vi "载荷控制(3).vi"() -> ()   [LabVIEW 2020]
doc: "The Basic Serial Read and Write example performs a Serial Port Read, a Serial Port Write, or a combination of these actions. The user selects the actions (read or write) on the front panel. If both are selected, the VI will write the data first, read data, and then close the VISA session that is opened to the port. This VI will wait until the specified number of bytes is received at the port. Only the number of bytes specified will be read.\n\nINSTRUCTIONS:\n1) Select the serial resource and configuration parameters (baud rate, data bits, parity, stop bits, flow control).\n2) Select the operations to be performed. \n3) Connect the serial port to your device. If no device is available, perform a loopback test by doing one of the following. Short pins 2 and 3 on a RS-232 cable or short pin 4 to pin 8 and pin 5 to pin 9 on a RS-485/422 cable. \n4) Run the VI to see the data read. (The \"read string\" will match the \"string to write\" if a loopback test was performed.)\n\nNote: The parameters set for the serial port must match the parameters of the connected instrument or device. In this example, the bytes to read parameter specifies the number of bytes that the serial port reads. If there were more bytes at the port than the number specified in bytes to read, those bytes would not be read. Also, if you specify to read more bytes than the number of bytes actually read, you might receive a timeout error message.\n\nOn the block diagram, the Configure Serial Port VI sets the configuration parameters. The front panel displays the controls used to configure the basic parameters, such as baud rate, data bits, and parity. Constants configure the other parameters the user probably does not need set. After the VISA Configure Serial Port VI opens the VISA session and configures the port, the VI passes the VISA resource name to other VIs that perform operations on that VISA resource. The VISA Write function sends a command to the serial device and the VISA Read function returns data based on the command. The VISA Close function then closes the reference to the serial device. It is important to close the reference; otherwise communication through with that port through protocols other than VISA might not be possible."
uses:
  <vilib>/Analysis/baseanly.llb/Mean (DBL).vi
  <vilib>/Instr/_visa.llb/VISA Configure Serial Port (Instr).vi
  <vilib>/Analysis/NI_AALBase.lvlib
panel:
  in  "停止 3":bool
  out "位移(微米）":dbl format="%#.2f"
  out "数据":dbl
  out "原始载荷":dbl format="%#.2f"
  out "当前次数":i32
  in  "选项卡控件":enum32{"设置", "手动", "自动", "循环加载"}(tab)
  in  "设置串口":refnum<visa-resource-name>="COM1"
  in  "载荷测量":tag="cDAQ9184-1ADFF13Mod3"
  in  "气流控制":tag="Dev2"
  in  "?":bool
  in  "?":bool
  in  "?":bool
  in  "?":bool
  in  "位置清零":bool
  in  "载荷清零":bool
  in  "加载":bool
  in  "比例系数":i32 min=0 max=1000
  in  "设定载荷":i32 min=0 max=1000
  in  "形变速率（微米/秒）":i32 min=0
  in  "火焰控制":dbl format="%#_6f"
  in  "冷却控制":dbl
  in  "开":bool
  in  "低载时间":dbl
  in  "高载时间":dbl
  in  "低载荷":dbl
  in  "高载荷":dbl
  in  "循环次数":i32
  out "载荷（牛）":dbl format="%.2f"
  out "载荷零点\n（牛）":dbl
  in  "停止":bool
  out "拉压":dbl
  in  "触发":u8
  out "结果":i16
  in  "实际位置":i32
  out "位移(微米）":dbl
  in  "停止 2":bool
  in  "自动\n\n手动":bool
  # "微调"
  # "粗调"
  # "关"
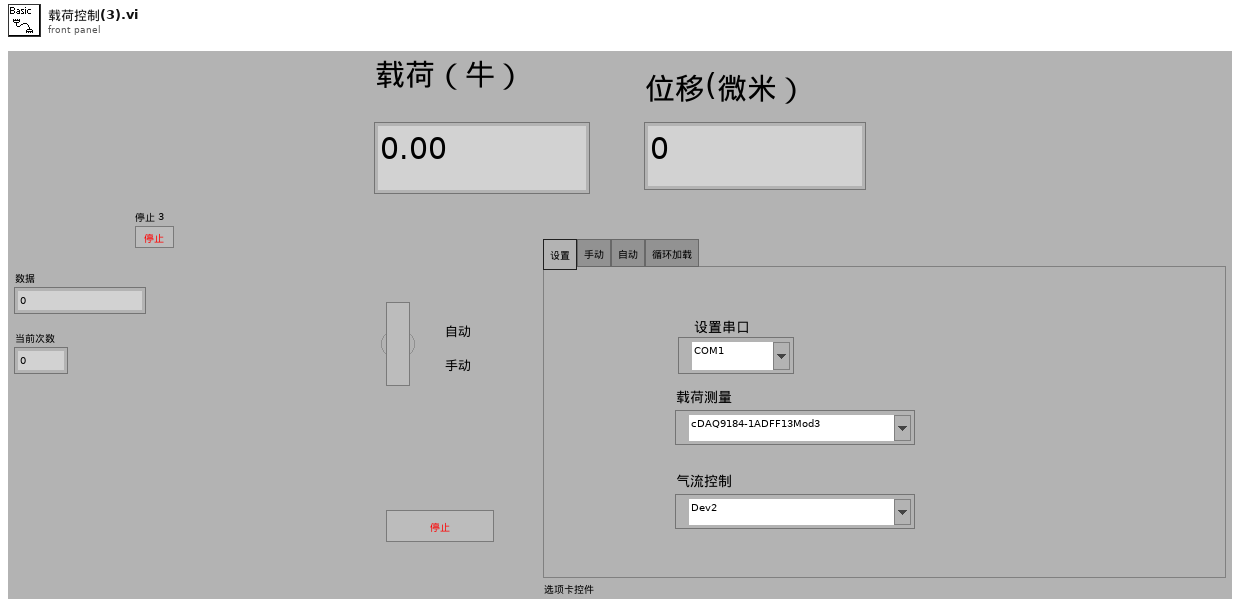
[diagram p1: front panel]
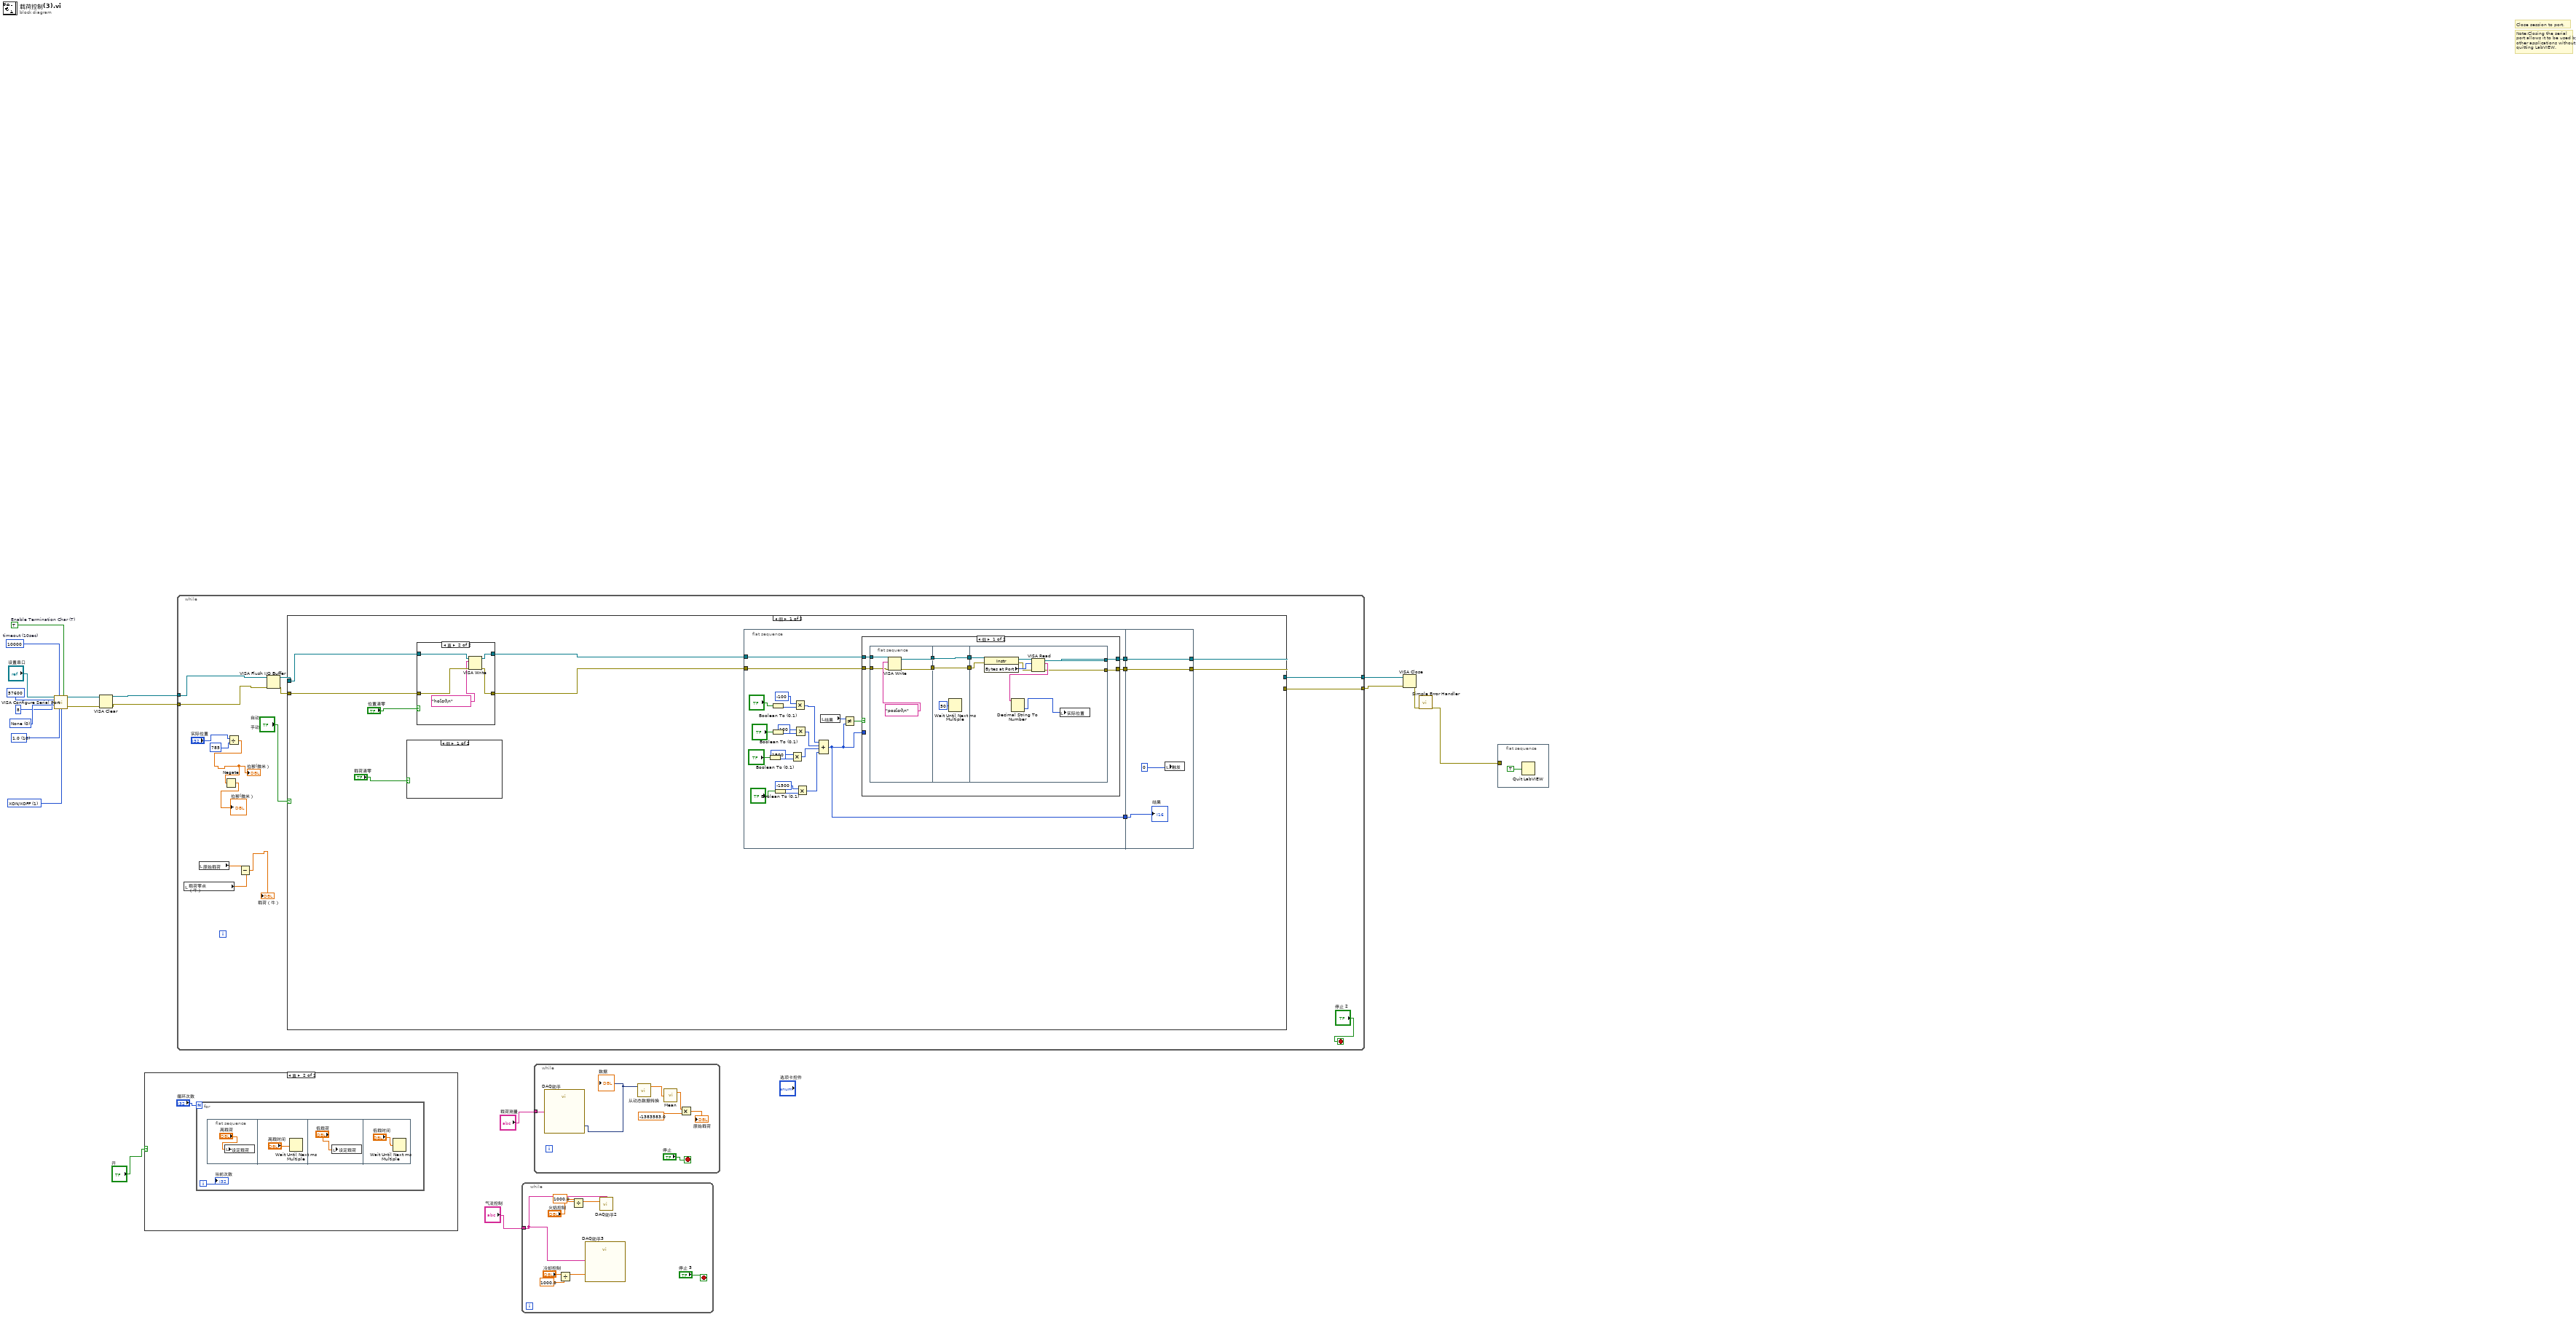
[diagram p0: block diagram]
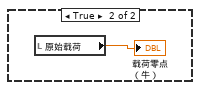
[diagram p3: hidden frame]
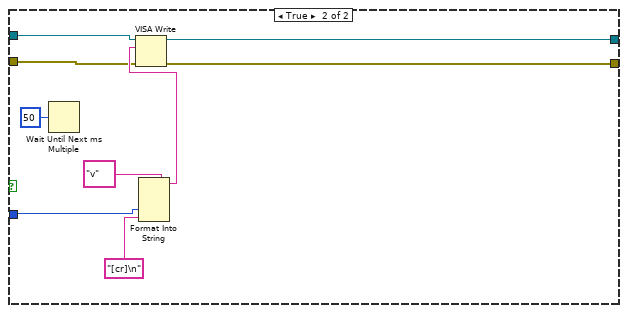
[diagram p5: hidden frame]
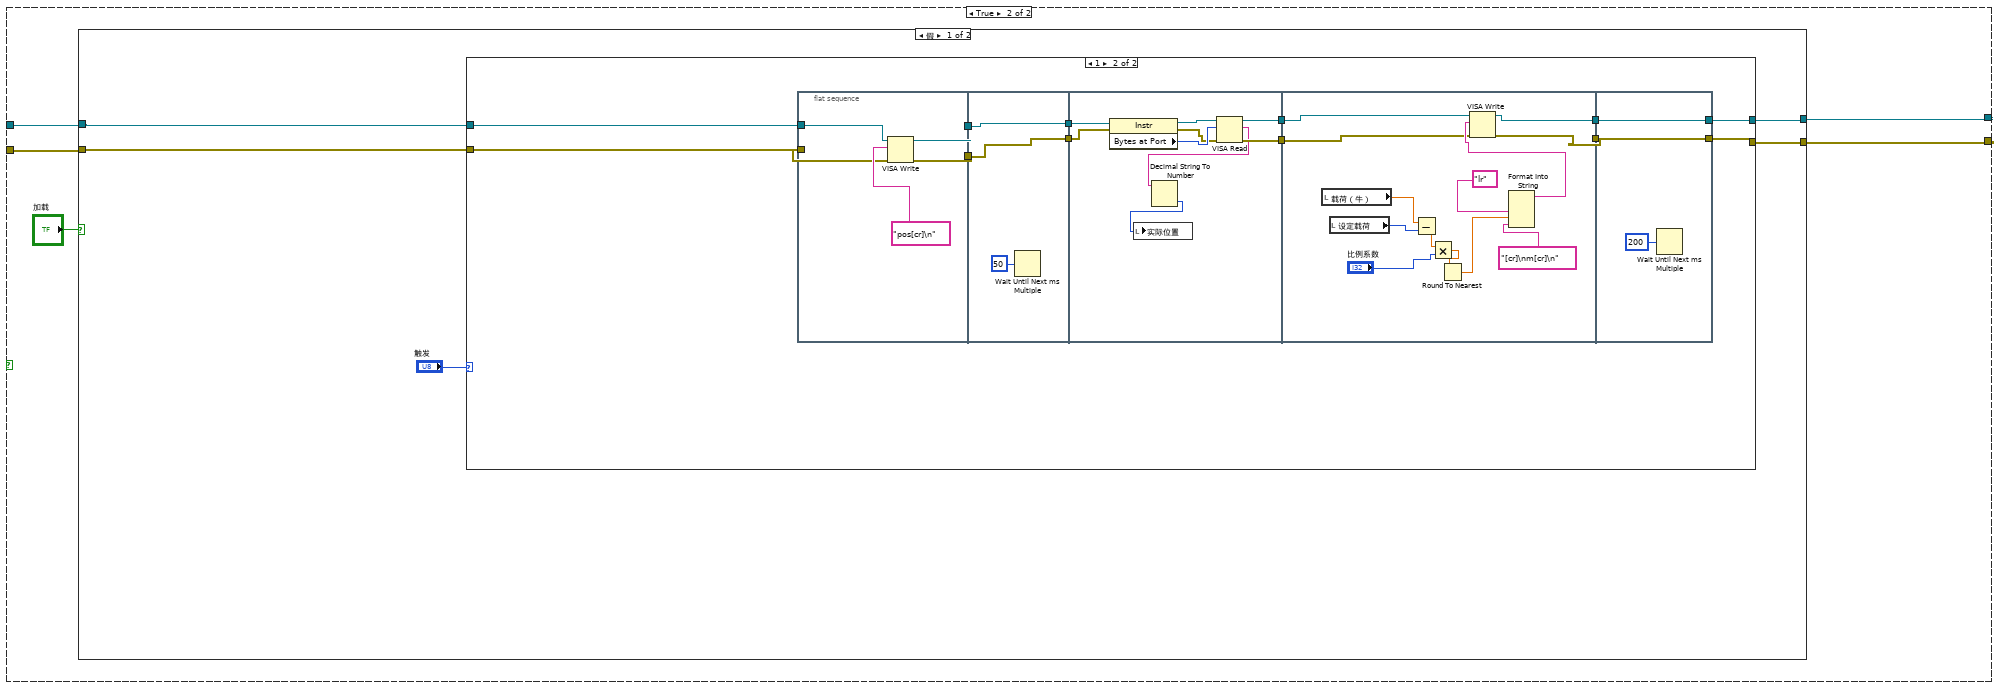
[diagram p6: hidden frame]
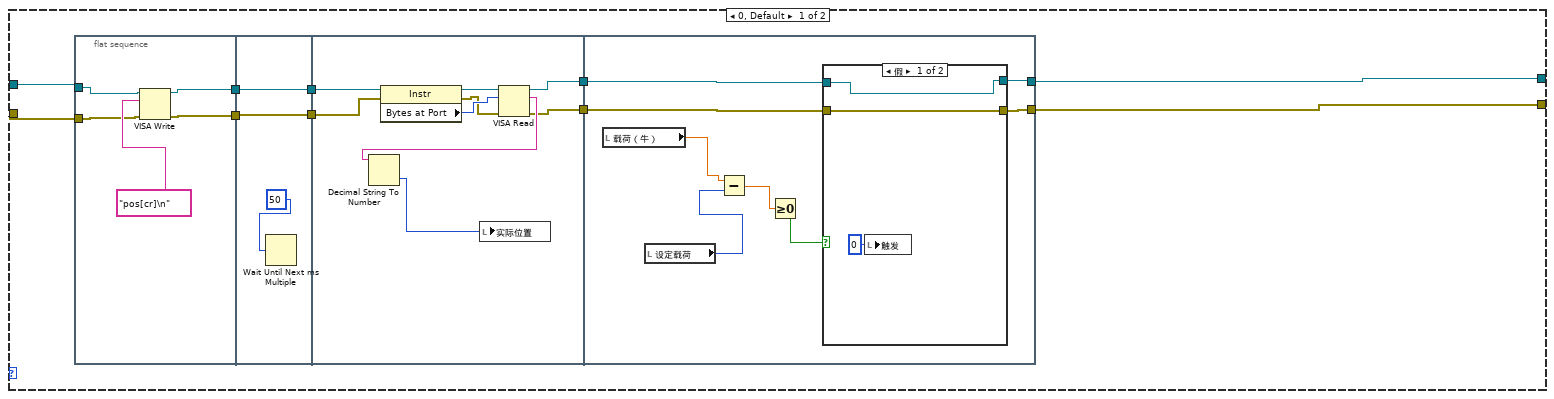
[diagram p7: hidden frame]
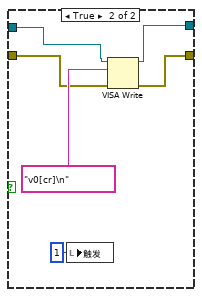
[diagram p8: hidden frame]
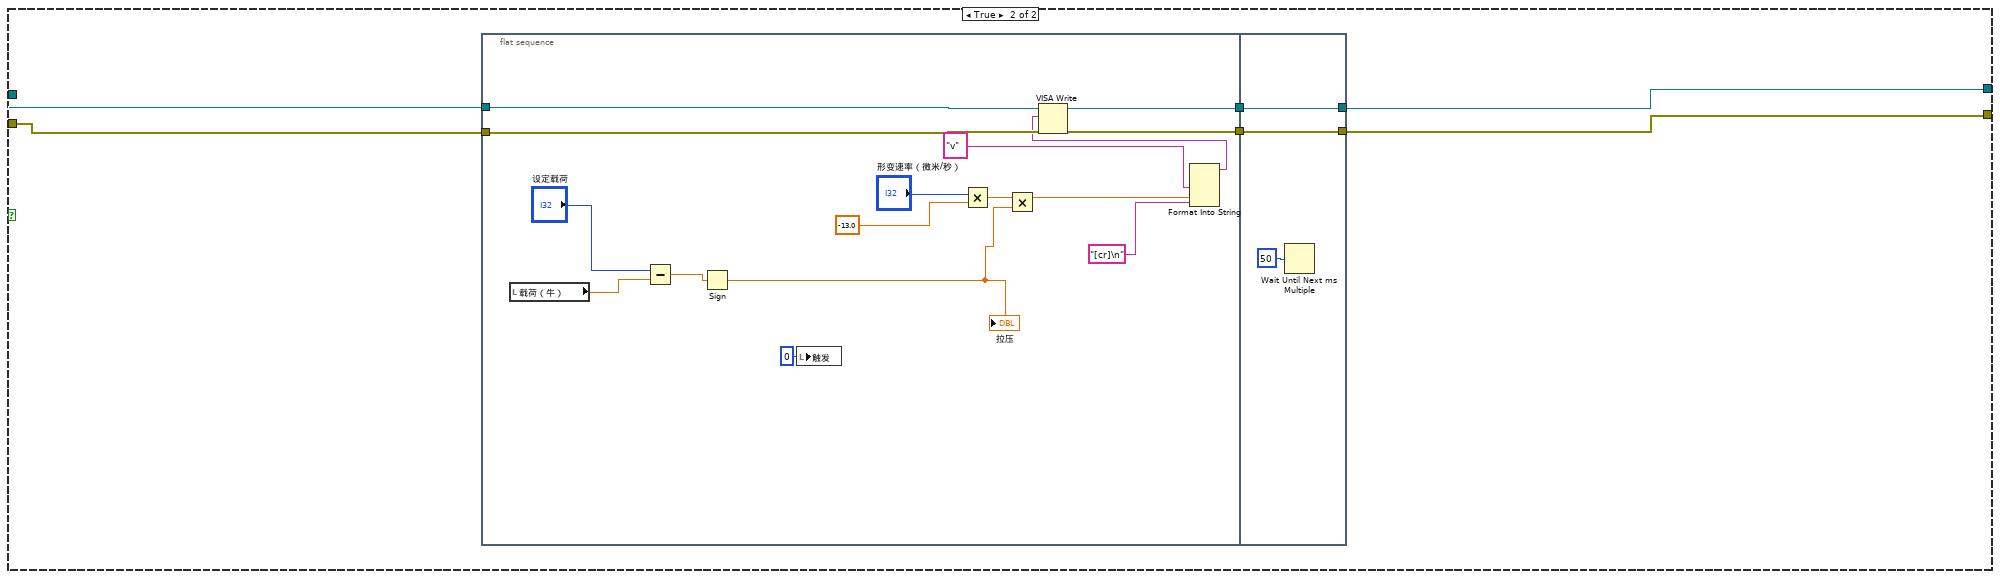
[diagram p9: hidden frame]
diagram:
  w13 = u16 1 items=["None"=0, "XON/XOFF"=1, "RTS/CTS"=2, "DTR/DSR"=4] ("flow control")
  w14 = u16 10 items=["1.0"=10, "1.5"=15, "2.0"=20] ("stop bits")
  w17 = u16 0 items=["None", "Odd", "Even", "Mark", "Space"] ("parity")
  w15 = TRUE  # Enable Termination Char (T)
  w16 = u32 10000  # timeout (10sec)
  # "Note:Closing the serial port allows it to be used by other applications without\nquitting LabVIEW."
  # "Close session to port."
  n1 = call-poly "VISA Configure Serial Port"("VISA resource name"="设置串口", "timeout (10sec)"=w16, "Enable Termination\nChar (T)"=w15, "baud rate (9600)"=u32 57600 ("baud rate"), "data bits (8)"=u16 8 ("data bits"), "parity (0:none)"=w17, "stop bits (10: 1 bit)"=w14, "flow control (0:none)"=w13) -> ("VISA resource name out"=w5:refnum<visa-resource-name>, "error out"=w7:errorcluster)  [unwired: 6 in]
  n2 = VISA Clear(VISA resource name=w5, error in (no error)=w7) -> (VISA resource name out=w6:refnum<visa-resource-name>, error out=w8:errorcluster)
  n3 = case shown="真" "开" {
    frame False {
    }
    frame True {
      n4 = for {
        N: "循环次数" -> [_]
        i -> [w21]
        n5 = flat-sequence {
          frame #0 {
            n6 = local write "设定载荷"("高载荷") -> ()
          }
          frame #1 {
            n7 = Wait Until Next ms Multiple(millisecond multiple="高载时间") -> ()  [unwired: 1 out]
          }
          frame #2 {
            n8 = local write "设定载荷"("低载荷") -> ()
          }
          frame #3 {
            n9 = Wait Until Next ms Multiple(millisecond multiple="低载时间") -> ()  [unwired: 1 out]
          }
        }
        "当前次数" <- w21
      }
    }
  }
  n10 = while {
    tunnel: w6 -> [w31]
    tunnel: w8 -> [w32]
    tunnel: [w38] -> w10
    tunnel: [w37] -> w9
    stop <- "停止 2" stop-if-true
    n11 = local read "载荷零点\n（牛）"() -> (w29:dbl)
    n12 = local read "原始载荷"() -> (w30:dbl)
    n13 = Divide(x="实际位置", y=785) -> (x/y=w26:dbl)
    "位移(微米）" <- w26
    n14 = Negate(x=w26) -> (-x=→"位移(微米）":dbl)
    n15 = Subtract(x=w30, y=w29) -> (x-y=→"载荷（牛）":dbl)
    n16 = VISA Flush I/O Buffer(VISA resource name=w31, error in (no error)=w32) -> (VISA resource name out=w34:refnum<visa-resource-name>, error out=w33:errorcluster)  [unwired: 1 in]
    n17 = case shown="假" "自动\n\n手动" {
      tunnel: w34 -> [w46 w125]
      tunnel: w33 -> [w44 w121]
      tunnel: [w48 w123] -> w38
      tunnel: [w47 w122] -> w37
      frame False {
        n18 = case shown="假" "载荷清零" {
          frame False {
          }
          frame True {
            n19 = local read "原始载荷"() -> (→"载荷零点\n（牛）":dbl)
          }
        }
        n20 = case shown="真" "位置清零" {
          tunnel: w46 -> [w54 w59]
          tunnel: [w54 w58] -> w45
          tunnel: w44 -> [w53 w57]
          tunnel: [w53 w56] -> w43
          frame False {
          }
          frame True {
            n21 = VISA Write(VISA resource name=w59, write buffer="ho[cr]\n" ("输入 1"), error in (no error)=w57) -> (VISA resource name out=w58:refnum<visa-resource-name>, error out=w56:errorcluster)  [unwired: 1 out]
          }
        }
        n22 = flat-sequence {
          tunnel: [w82] -> w51
          tunnel: [w69] -> w49
          tunnel: [w68] -> w50
          tunnel: w45 -> [w65]
          tunnel: w43 -> [w66]
          tunnel: w51 -> [w119]
          tunnel: w50 -> [w120]
          tunnel: w49 -> [w118]
          tunnel: [w119] -> w48
          tunnel: [w118] -> w47
          frame #0 {
            n23 = Boolean To (0,1)(Boolean="?") -> (0, 1=w62:i16)
            n24 = Boolean To (0,1)(Boolean="?") -> (0, 1=w80:i16)
            n25 = Boolean To (0,1)(Boolean="?") -> (0, 1=w78:i16)
            n26 = Boolean To (0,1)(Boolean="?") -> (0, 1=w76:i16)
            n27 = Multiply(x=i16 1500, y=w62) -> (x*y=w60:i16)
            n28 = Multiply(x=i16 -100, y=w80) -> (x*y=w73:i16)
            n29 = Multiply(x=i16 100, y=w78) -> (x*y=w72:i16)
            n30 = Multiply(x=i16 -1500, y=w76) -> (x*y=w71:i16)
            n31 = Compound Arithmetic op=ADD(w73, w72, w60, w71) -> (w68:i16)
            n32 = local read "结果"() -> (w67:i16)
            n33 = Not Equal?(x=w67, y=w68) -> (x != y?=w70:bool)
            n34 = case shown="假" w70 {
              tunnel: w65 -> [w86 w110]
              tunnel: [w90 w113] -> w82
              tunnel: w68 -> [_ w112]
              tunnel: w66 -> [w85 w109]
              tunnel: [w87 w111] -> w69
              frame False {
                n35 = flat-sequence {
                  tunnel: [w92] -> w89
                  tunnel: [w91] -> w88
                  tunnel: w86 -> [w94]
                  tunnel: w85 -> [w93]
                  tunnel: w89 -> [w97]
                  tunnel: w88 -> [w96]
                  tunnel: [w97] -> w84
                  tunnel: [w96] -> w83
                  tunnel: [w104] -> w90
                  tunnel: [w102] -> w87
                  tunnel: w84 -> [w101]
                  tunnel: w83 -> [w100]
                  frame #0 {
                    n36 = VISA Write(VISA resource name=w94, write buffer="pos[cr]\n" ("输入 1"), error in (no error)=w93) -> (VISA resource name out=w92:refnum<visa-resource-name>, error out=w91:errorcluster)  [unwired: 1 out]
                  }
                  frame #1 {
                    n37 = Wait Until Next ms Multiple(millisecond multiple=u32 50 ("毫秒倍数")) -> ()  [unwired: 1 out]
                  }
                  frame #2 {
                    n38 = property class="Instr"(reference=w101, error in=w100) -> (reference out=w105:refnum<visa-resource-name>, error out=w103:errorcluster, "Bytes at Port"=w106:u32)
                    n39 = VISA Read(VISA resource name=w105, byte count=w106, error in (no error)=w103) -> (VISA resource name out=w104:refnum<visa-resource-name>, read buffer=w107:string, error out=w102:errorcluster)  [unwired: 1 out]
                    n40 = Decimal String To Number(string=w107) -> (number=w99:i32)  [unwired: 2 in, 1 out]
                    n41 = local write "实际位置"(w99) -> ()
                  }
                }
              }
              frame True {
                n42 = Wait Until Next ms Multiple(millisecond multiple=u32 50 ("毫秒倍数")) -> ()  [unwired: 1 out]
                n43 = Format Into String("v" ("输入 1"), w112, "[cr]\n" ("输入 3")) -> (resulting string=w114:string)  [unwired: 3 in, 1 out]
                n44 = VISA Write(VISA resource name=w110, write buffer=w114, error in (no error)=w109) -> (VISA resource name out=w113:refnum<visa-resource-name>, error out=w111:errorcluster)  [unwired: 1 out]
              }
            }
          }
          frame #1 {
            n45 = local write "触发"(u8 0 ("触发")) -> ()
            "结果" <- w120
          }
        }
      }
      frame True {
        n46 = case shown="假" "加载" {
          tunnel: w125 -> [w129 w225]
          tunnel: w121 -> [w128 w224]
          tunnel: [w127 w223] -> w123
          tunnel: [w130 w222] -> w122
          frame False {
            n47 = case shown="1" "触发" {
              tunnel: [w136 w179] -> w130
              tunnel: w129 -> [w135 w182]
              tunnel: w128 -> [w134 w181]
              tunnel: [w131 w180] -> w127
              frame 0, Default {
                n48 = flat-sequence {
                  tunnel: [w145] -> w140
                  tunnel: [w144] -> w139
                  tunnel: w134 -> [w141]
                  tunnel: w135 -> [w142]
                  tunnel: [w148] -> w138
                  tunnel: w140 -> [w148]
                  tunnel: [w147] -> w137
                  tunnel: w139 -> [w147]
                  tunnel: w138 -> [w157]
                  tunnel: w137 -> [w155]
                  tunnel: [w151] -> w133
                  tunnel: [w150] -> w132
                  tunnel: [w162] -> w131
                  tunnel: [w165] -> w136
                  tunnel: w133 -> [w164]
                  tunnel: w132 -> [w163]
                  frame #0 {
                    n49 = VISA Write(VISA resource name=w142, write buffer="pos[cr]\n" ("输入 1"), error in (no error)=w141) -> (VISA resource name out=w145:refnum<visa-resource-name>, error out=w144:errorcluster)  [unwired: 1 out]
                  }
                  frame #1 {
                    n50 = Wait Until Next ms Multiple(millisecond multiple=u32 50 ("等待时间（毫秒）")) -> ()  [unwired: 1 out]
                  }
                  frame #2 {
                    n51 = property class="Instr"(reference=w157, error in=w155) -> (reference out=w156:refnum<visa-resource-name>, error out=w152:errorcluster, "Bytes at Port"=w153:u32)
                    n52 = VISA Read(VISA resource name=w156, byte count=w153, error in (no error)=w152) -> (VISA resource name out=w150:refnum<visa-resource-name>, read buffer=w154:string, error out=w151:errorcluster)  [unwired: 1 out]
                    n53 = Decimal String To Number(string=w154) -> (number=w149:i32)  [unwired: 2 in, 1 out]
                    n54 = local write "实际位置"(w149) -> ()
                  }
                  frame #3 {
                    n55 = local read "载荷（牛）"() -> (w159:dbl)
                    n56 = local read "设定载荷"() -> (w161:i32)
                    n57 = Subtract(x=w159, y=w161) -> (x-y=w158:dbl)
                    n58 = Greater Or Equal To 0?(x=w158) -> (x >= 0?=w160:bool)
                    n59 = case shown="假" w160 {
                      tunnel: [w167 w172] -> w165
                      tunnel: [w166 w171] -> w162
                      tunnel: w164 -> [w167 w169]
                      tunnel: w163 -> [w166 w170]
                      frame False {
                        n60 = local write "触发"(u8 0 ("触发")) -> ()
                      }
                      frame True {
                        n61 = local write "触发"(u8 1 ("触发")) -> ()
                        n62 = VISA Write(VISA resource name=w170, write buffer="v0[cr]\n" ("输入 1"), error in (no error)=w169) -> (VISA resource name out=w171:refnum<visa-resource-name>, error out=w172:errorcluster)  [unwired: 1 out]
                      }
                    }
                  }
                }
              }
              frame 1 {
                n63 = flat-sequence {
                  tunnel: [w190] -> w185
                  tunnel: [w189] -> w183
                  tunnel: w181 -> [w188]
                  tunnel: w182 -> [w187]
                  tunnel: [w194] -> w186
                  tunnel: w185 -> [w194]
                  tunnel: [w193] -> w184
                  tunnel: w183 -> [w193]
                  tunnel: w184 -> [w196]
                  tunnel: w186 -> [w197]
                  tunnel: [w203] -> w178
                  tunnel: [w202] -> w177
                  tunnel: [w213] -> w176
                  tunnel: [w214] -> w175
                  tunnel: w177 -> [w211]
                  tunnel: w178 -> [w210]
                  tunnel: [w218] -> w179
                  tunnel: [w219] -> w180
                  tunnel: w176 -> [w219]
                  tunnel: w175 -> [w218]
                  frame #0 {
                    n64 = VISA Write(VISA resource name=w187, write buffer="pos[cr]\n" ("输入 1"), error in (no error)=w188) -> (VISA resource name out=w190:refnum<visa-resource-name>, error out=w189:errorcluster)  [unwired: 1 out]
                  }
                  frame #1 {
                    n65 = Wait Until Next ms Multiple(millisecond multiple=u32 50 ("毫秒倍数")) -> ()  [unwired: 1 out]
                  }
                  frame #2 {
                    n66 = property class="Instr"(reference=w197, error in=w196) -> (reference out=w201:refnum<visa-resource-name>, error out=w198:errorcluster, "Bytes at Port"=w199:u32)
                    n67 = VISA Read(VISA resource name=w201, byte count=w199, error in (no error)=w198) -> (VISA resource name out=w203:refnum<visa-resource-name>, read buffer=w200:string, error out=w202:errorcluster)  [unwired: 1 out]
                    n68 = Decimal String To Number(string=w200) -> (number=w195:i32)  [unwired: 2 in, 1 out]
                    n69 = local write "实际位置"(w195) -> ()
                  }
                  frame #3 {
                    n70 = local read "载荷（牛）"() -> (w209:dbl)
                    n71 = local read "设定载荷"() -> (w208:i32)
                    n72 = Subtract(x=w209, y=w208) -> (x-y=w207:dbl)
                    n73 = Multiply(x=w207, y="比例系数") -> (x*y=w205:dbl)
                    n74 = Round To Nearest(number=w205) -> (nearest integer value=w204:dbl)
                    n75 = Format Into String("lr" ("输入 1"), w204, "[cr]\nm[cr]\n" ("输入 3")) -> (resulting string=w212:string)  [unwired: 3 in, 1 out]
                    n76 = VISA Write(VISA resource name=w210, write buffer=w212, error in (no error)=w211) -> (VISA resource name out=w213:refnum<visa-resource-name>, error out=w214:errorcluster)  [unwired: 1 out]
                  }
                  frame #4 {
                    n77 = Wait Until Next ms Multiple(millisecond multiple=u32 200 ("毫秒倍数")) -> ()  [unwired: 1 out]
                  }
                }
              }
            }
          }
          frame True {
            n78 = flat-sequence {
              tunnel: w225 -> [w241]
              tunnel: w224 -> [w240]
              tunnel: [w239] -> w221
              tunnel: [w238] -> w220
              tunnel: [w243] -> w222
              tunnel: [w244] -> w223
              tunnel: w221 -> [w244]
              tunnel: w220 -> [w243]
              frame #0 {
                n79 = local read "载荷（牛）"() -> (w229:dbl)
                n80 = Subtract(x="设定载荷", y=w229) -> (x-y=w228:dbl)
                n81 = Sign(1:w228) -> (0:w226:dbl)
                "拉压" <- w226
                n82 = local write "触发"(u8 0 ("触发")) -> ()
                n83 = Multiply(x="形变速率（微米/秒）", y=-13.0 ("x")) -> (x*y=w233:dbl)
                n84 = Multiply(x=w233, y=w226) -> (x*y=w227:dbl)
                n85 = Format Into String("v" ("输入 1"), w227, "[cr]\n" ("输入 3")) -> (resulting string=w235:string)  [unwired: 3 in, 1 out]
                n86 = VISA Write(VISA resource name=w241, write buffer=w235, error in (no error)=w240) -> (VISA resource name out=w239:refnum<visa-resource-name>, error out=w238:errorcluster)  [unwired: 1 out]
              }
              frame #1 {
                n87 = Wait Until Next ms Multiple(millisecond multiple=u32 50 ("毫秒倍数")) -> ()  [unwired: 1 out]
              }
            }
          }
        }
      }
    }
  }
  n88 = while {
    tunnel: "气流控制" -> [w251]
    stop <- "停止 3" stop-if-true
    n89 = Divide(x="冷却控制", y=1000.0) -> (x/y=w246:dbl)
    n90 = Divide(x="火焰控制", y=1000.0) -> (x/y=w248:dbl)
    n91 = call "DAQ助手3"("data"=w246, "设备名"=w251) -> ()  [unwired: 16 in, 2 out]
    n92 = call "DAQ助手2"("data"=w248, "设备名"=w251) -> ()  [unwired: 16 in, 2 out]
  }
  n93 = while {
    tunnel: "载荷测量" -> [w253]
    stop <- "停止" stop-if-true
    n94 = call "DAQ助手"("设备名"=w253) -> ("data"=w255:dynamicdata)  [unwired: 16 in, 2 out]
    "数据" <- w255
    n95 = call "从动态数据转换"("Dynamic Data Type"=w255) -> ("Array"=w256:dbl[])  [unwired: 3 in]
    n96 = call-poly <vilib>:"Mean.vi"("X"=w256) -> ("mean"=w254:dbl)  [unwired: 1 out]
    n97 = Multiply(x=w254, y=-1383583.0) -> (x*y=→"原始载荷":dbl)
  }
  n98 = VISA Close(VISA resource name=w10, error in (no error)=w9) -> (error out=w18:errorcluster)
  n99 = call <vilib>:"Simple Error Handler.vi"("error in (no error)"=w18) -> ("error out"=w4:errorcluster)  [unwired: 4 in, 4 out]
  n100 = flat-sequence {
    tunnel: w4 -> [_]
    frame #0 {
      n101 = Quit LabVIEW(quit? (T)=TRUE ("退出？(T)")) -> ()
    }
  }
